vi "LVClass_ClosedLoopSecurityActivation Read ClosedLoopSecurityActivation ptr.vi"(8 "error in (no error)":errorcluster, 11 "ClosedLoopSecurityActivation in":refnum<class "ClosedLoopSecurityActivation.lvclass">) -> (0 "error out":errorcluster, 2 "ClosedLoopSecurityActivation":T1, 3 "ClosedLoopSecurityActivation out":refnum<class "ClosedLoopSecurityActivation.lvclass">)   [LabVIEW 2020, in "ClosedLoopSecurityActivation.lvclass"]
uses:
  ClosedLoopSecurityActivation.lvclass
  Controls/ClassID.ctl
  ClosedLoopSecurityActivation.lvclass/ClosedLoopSecurityActivation.ctl
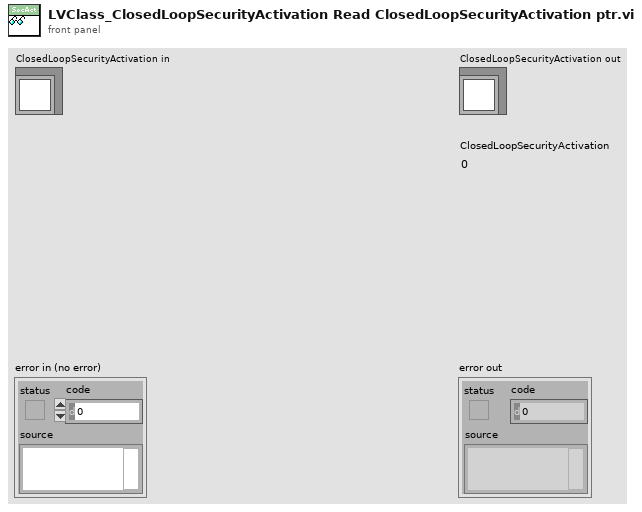
[diagram p1: front panel]
types:
  T1 = typedef "ClassID.ctl" = i64
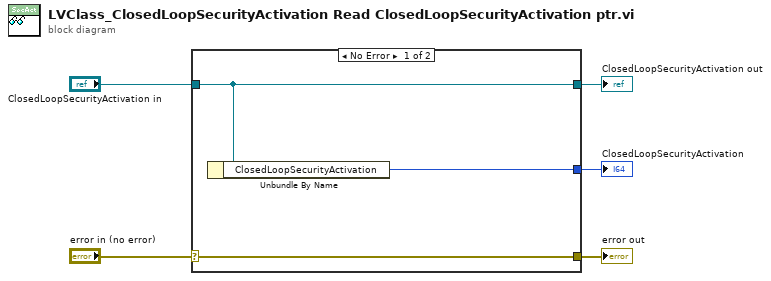
[diagram p0: block diagram]
diagram:
  n1 = case shown="No Error" "error in (no error)" {
    selector: "error in (no error)" -> [w8 w9]
    tunnel: [w8 w9] -> w4
    tunnel: [w7 w10] -> w2
    tunnel: "ClosedLoopSecurityActivation in" -> [w7 w10]
    tunnel: [w6 _] -> w1
    frame No Error {
      n2 = Unbundle By Name(w7) -> ("ClosedLoopSecurityActivation"=w6:T1)
    }
    frame Error {
    }
  }
  "error out" <- w4
  "ClosedLoopSecurityActivation out" <- w2
  "ClosedLoopSecurityActivation" <- w1
